vi "decodeUint32.vi"(8 "error in (no error)":errorcluster, 11 "ByteArray":u8[](array[numeric]) format="%x") -> (0 "error out":errorcluster, 1 "Uint32":u32, 2 "Variant":variant, 3 "RemainingBytes":u8[](array[numeric]) format="%x", 5 "Type":string)   [LabVIEW 2015, in "MsgPack.lvlib"]
uses:
  MsgPack.lvlib
  <vilib>/ErrorRing/Error Ring.xnode
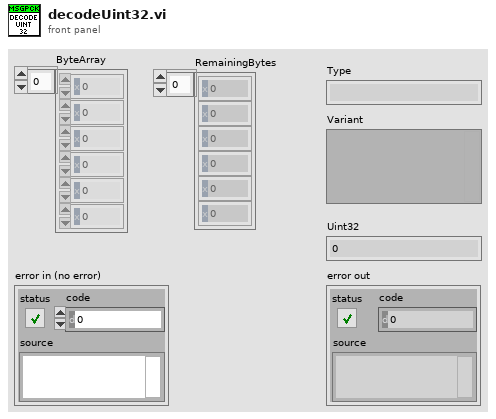
[diagram p1: front panel]
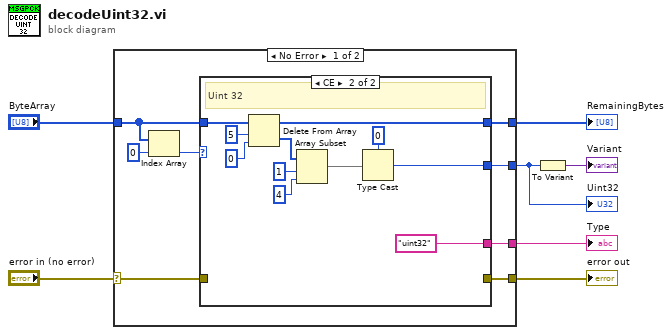
[diagram p0: block diagram]
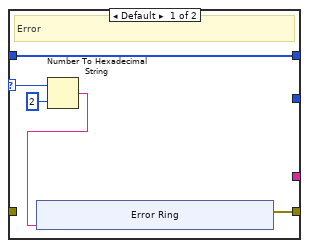
[diagram p2: hidden frame]
diagram:
  n1 = case shown="No Error" "error in (no error)" {
    selector: "error in (no error)" -> [w12 w38]
    tunnel: [w15 w38] -> w6
    tunnel: [w14 _] -> w5
    tunnel: [w13 _] -> w4
    tunnel: "ByteArray" -> [w10 w37]
    tunnel: [w11 w37] -> w2
    frame No Error {
      n2 = Index Array(array=w10, index=0) -> (element=w9:u8)
      n3 = case shown="CE" w9 {
        selector: w9 -> [w17 _]
        tunnel: [w19 _] -> w15
        tunnel: w12 -> [_ _]
        tunnel: [_ "uint32"] -> w14
        tunnel: [_ w26] -> w13
        tunnel: [w20 w33] -> w11
        tunnel: w10 -> [w20 w34]
        frame Default {
          # "Error"
          n4 = Number To Hexadecimal String(1:i16 2 ("width (-)"), 2:w17) -> (0:w16:string)
          n5 = xnode "Error Ring"("parameter 0"=w16) -> ("error out"=w19:errorcluster)
        }
        frame 206 {
          # "Uint 32"
          n6 = Delete From Array(array=w34, length=5, index=0) -> (deleted portion=w27:u8[], array with subset deleted=w33:u8[])
          n7 = Array Subset(array=w27, index=1, length=4) -> (w30:u8[])
          n8 = Type Cast(type=u32 0, x=w30) -> (*(type *) &x=w26:u32)
        }
      }
    }
    frame Error {
    }
  }
  "error out" <- w6
  "Type" <- w5
  "Uint32" <- w4
  "RemainingBytes" <- w2
  n9 = To Variant(anything=w4) -> (Variant=→"Variant":variant)
